vi "get freq ring.vi"(8 "error in (no error)":errorcluster caption="에러 입력(에러 없음)", 11 "DW7912 입력":refnum<class "DW7912.lvclass">) -> (0 "error out":errorcluster caption="에러 출력", 1 "caption":string="PWM", 2 "strings & values":T1=[{"String"="24kHz", "Value"=24000}, {"String"="48kHz", "Value"=48000}, {"String"="96kHz", "Value"=96000}, {"String"="12kHz", "Value"=12000}], 3 "DW7912 출력":refnum<class "DW7912.lvclass">, 4 "read value":u32)   [LabVIEW 2020, in "DW7912.lvclass"]
uses:
  DW7912.lvclass
  <vilib>/Utility/miscctls.llb/LVStringsAndValuesArrayTypeDef_U32.ctl
  Haptic IC/Haptic IC.lvclass/Haptic IC.ctl
  SubVIs/I2C/Instance VIs/(SubVI)I2C_8Bit-8Bit_Read_Single.vi
  Haptic IC/Haptic IC.lvclass
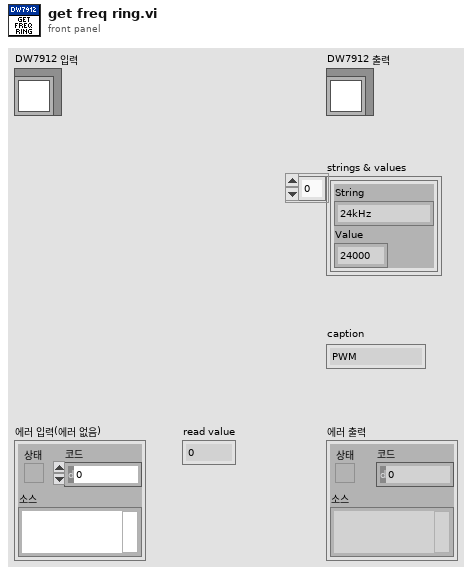
[diagram p1: front panel]
types:
  T1 = typedef "LVStringsAndValuesArrayTypeDef_U32.ctl" = cluster{"String":string, "Value":u32}[]
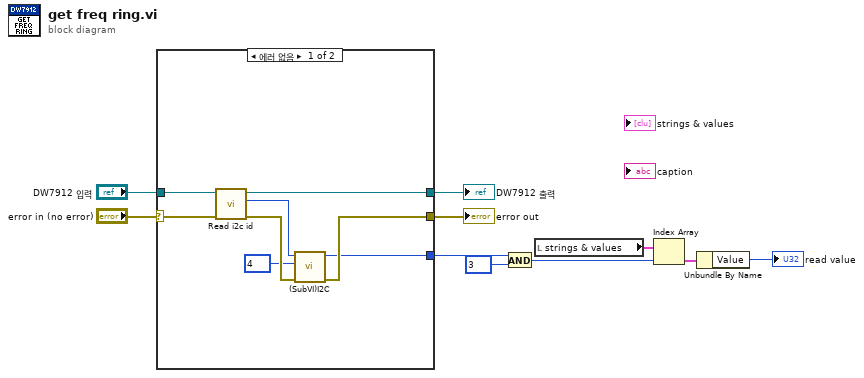
[diagram p0: block diagram]
diagram:
  n1 = case shown="에러 없음" "error in (no error)" {
    selector: "error in (no error)" -> [w17 w19]
    tunnel: "DW7912 입력" -> [w18 w20]
    tunnel: [w16 w20] -> w4
    tunnel: [w12 w19] -> w5
    tunnel: [w11 _] -> w8
    frame No Error {
      n2 = call "Read i2c id.vi"("error in (no error)"=w17, "Haptic IC 입력"=w18) -> ("error out"=w15:errorcluster, "i2c id"=w14:u8, "Haptic IC 출력"=w16:refnum<class "DW7912.lvclass">)  [unwired: 7 in]
      n3 = call-poly "(SubVI)I2C.vi"("error in (no error)"=w15, "Address"=u8 4, "ID"=w14) -> ("error out"=w12:errorcluster, "Read Data"=w11:u8)  [unwired: 6 in, 1 out]
    }
    frame Error {
    }
  }
  "error out" <- w5
  "DW7912 출력" <- w4
  n4 = And(x=w8, y=u8 3) -> (x .and. y?=w3:u8)
  n5 = local read "strings & values"() -> (w9:T1)
  n6 = Index Array(array=w9, index=w3) -> (element=w10:cluster{"String":string, "Value":u32})
  n7 = Unbundle By Name(w10) -> ("Value"=→"read value":u32)
